vi "WPI_MXP_ChannelCache.vi"(7 "Shared MXP Pin":T1, 9 "Operation":T2, 11 "error in (no error)":errorcluster) -> (6 "Allocated?":bool, 15 "error out":errorcluster)   [LabVIEW 2017]
doc: "This software is licensed. Open the labview\\readme\\WPI Robotics Library Open Source License.txt file for more information."
uses:
  <vilib>/Rock Robotics/WPI/PWM/WPI_PWMChannelCacheOp.ctl
  <vilib>/Rock Robotics/WPI/MXP/WPI_MXP Shared MXP Pin.ctl
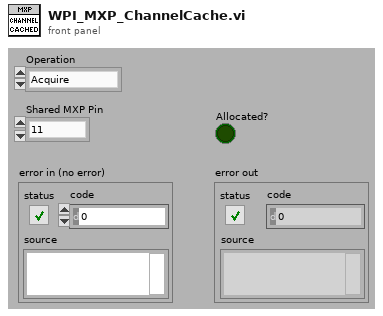
[diagram p1: front panel]
types:
  T1 = typedef "WPI_MXP Shared MXP Pin.ctl" = enum16{"11", "13", "15", "17", "19", "21", "23", "25", "27", "29", "31", "18", "22", "26", "32", "34", "Invalid"}
  T2 = typedef "WPI_PWMChannelCacheOp.ctl" = enum16{"Acquire", "Release", "Status"}
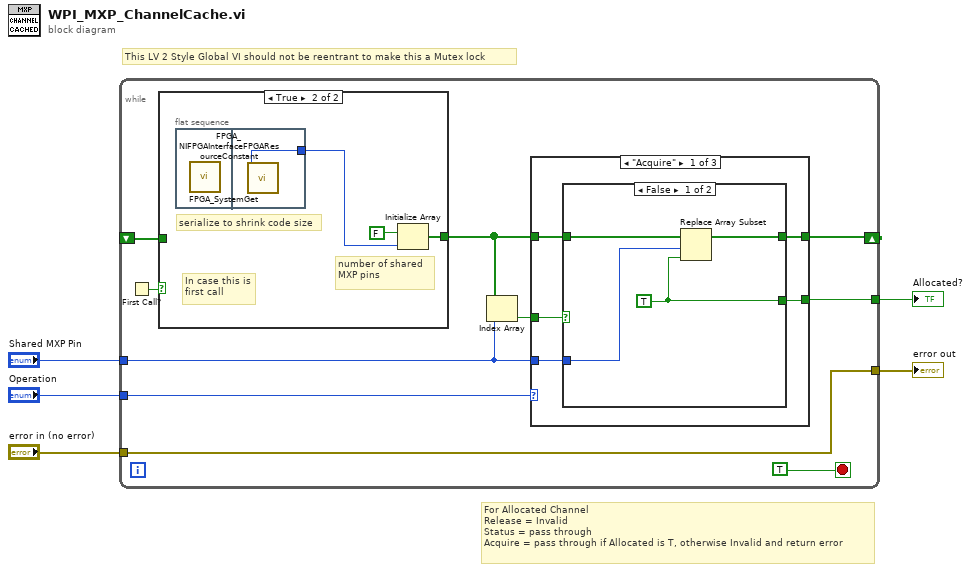
[diagram p0: block diagram]
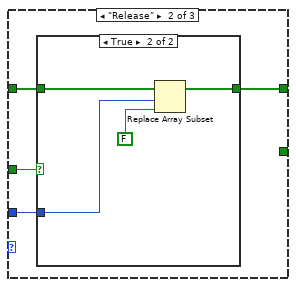
[diagram p3: hidden frame]
diagram:
  # "For Allocated Channel\nRelease = Invalid\nStatus = pass through\nAcquire = pass through if Allocated is T, otherwise Invalid and return error"
  # "This LV 2 Style Global VI should not be reentrant to make this a Mutex lock"
  n1 = while {
    shift-right: [w12] -> _
    shift-left: _ -> [w14]
    tunnel: "Operation" -> [w13]
    tunnel: "Shared MXP Pin" -> [w6]
    tunnel: [w8] -> w3
    tunnel: [w11] -> w2
    tunnel: "error in (no error)" -> [w8]
    stop <- TRUE stop-if-true
    n2 = First Call?() -> (First Call?: T/F=w15:bool)
    n3 = case shown="True" w15 {
      tunnel: w14 -> [w37 _]
      tunnel: [w37 w39] -> w7
      frame False {
      }
      frame True {
        # "number of shared MXP pins"
        # "serialize to shrink code size"
        # "In case this is\nfirst call"
        n4 = flat-sequence {
          tunnel: [w41] -> w38
          frame #0 {
            n5 = call <vilib>:"FPGA_SystemGet.vi"() -> ()  [unwired: 2 in, 10 out]
          }
          frame #1 {
            n6 = call <vilib>:"FPGA_NIFPGAInterfaceFPGAResourceConstant.vi"() -> ("NumberOfSharedMXPpins"=w41:u32)  [unwired: 11 out]
          }
        }
        n7 = Initialize Array(FALSE, w38) -> (w39:bool[])
      }
    }
    n8 = Index Array(array=w7, index=w6) -> (element=w9:bool)
    n9 = case shown="\"Acquire\"" w13 {
      tunnel: w7 -> [w17 w29 w35]
      tunnel: [w20 w27 w35] -> w12
      tunnel: w6 -> [w19 w28 _]
      tunnel: [w18 _ w36] -> w11
      tunnel: w9 -> [w16 w26 w36]
      frame "Acquire" {
        n10 = case shown="False" w16 {
          tunnel: w17 -> [w23 w25]
          tunnel: [w22 w25] -> w20
          tunnel: w19 -> [w21 _]
          tunnel: [w24 _] -> w18
          frame False {
            w24 = TRUE ("new element/subarray")
            n11 = Replace Array Subset(array=w23, new element=w24, index=w21) -> (w22:bool[])
          }
          frame True {
          }
        }
      }
      frame "Release" {
        n12 = case shown="True" w26 {
          tunnel: w29 -> [w30 w34]
          tunnel: w28 -> [_ w33]
          tunnel: [w30 w32] -> w27
          frame False {
          }
          frame True {
            n13 = Replace Array Subset(array=w34, new element=FALSE ("new element/subarray"), index=w33) -> (w32:bool[])
          }
        }
      }
      frame "Status" {
      }
    }
  }
  "error out" <- w3
  "Allocated?" <- w2
